vi "AdaptiveThreshold.vi"(4 "Kernel Block Size (Default: 5)":T1=enum."5", 5 "Adaptive Threshold Method":T2, 6 "Invert? (Default: False)":bool, 7 "Max Value (Default: 255)":u8=255, 8 "error in (no error)":errorcluster, 9 "C":dbl, 10 "Adaptive Threshold Result in":T3, 11 "Greyscale Image-Source in":T3) -> (0 "error out":errorcluster, 3 "Adaptive Threshold Result":T3)   [LabVIEW 2020, in "image.lvlib"]
doc: "Apply an adaptive threshold to convert a greyscale image to a binary image."
uses:
  image.lvlib
  Greyscale Image.ctl
  AdaptiveThresholdMethod.ctl
  Kernel Block Size.ctl
  common/common.lvlib
  common/bin/gartoolkit_32-1.dll
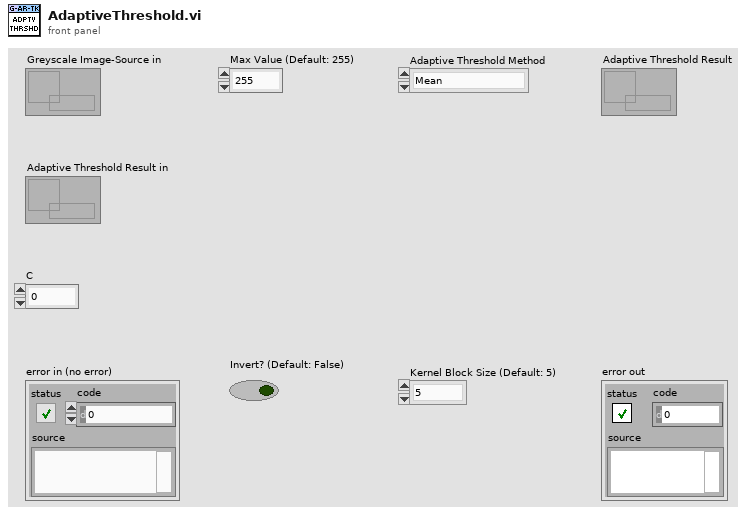
[diagram p1: front panel]
types:
  T1 = typedef "image.lvlib/Kernel Block Size.ctl" = enum16{"3", "5", "7", "9", "11", "13", "15", "17", "19", "21", "23", "25", "27", "29", "31", "33", "35", "37", "39", "41", "43", "45", "47", "49", "51", "53", "55", "57", "59", "61", "63", "65", "67", "69", "71", "73", "75", "77", "79", "81", "83", "85", "87", "89", "91", "93", "95", "97", "99", "101", "103", "105", "107", "109", "111", "113", "115", "117", "119", "121", "123", "125", "127", "129", "131", "133", "135", "137", "139", "141", "143", "145", "147", "149", "151", "153", "155", "157", "159", "161", "163", "165", "167", "169", "171", "173", "175", "177", "179", "181", "183", "185", "187", "189", "191", "193", "195", "197", "199", "201", "203", "205", "207", "209", "211", "213", "215", "217", "219", "221", "223", "225", "227", "229", "231", "233", "235", "237", "239", "241", "243", "245", "247", "249", "251", "253", "255", "257", "259", "261", "263", "265", "267", "269", "271", "273", "275", "277", "279", "281", "283", "285", "287", "289", "291", "293", "295", "297", "299", "301", "303", "305", "307", "309", "311", "313", "315", "317", "319", "321", "323", "325", "327", "329", "331", "333", "335", "337", "339", "341", "343", "345", "347", "349", "351", "353", "355", "357"}
  T2 = typedef "image.lvlib/AdaptiveThresholdMethod.ctl" = enum8{"Mean", "Gaussian"}
  T3 = typedef "image.lvlib/Greyscale Image.ctl" = refnum<data-value>
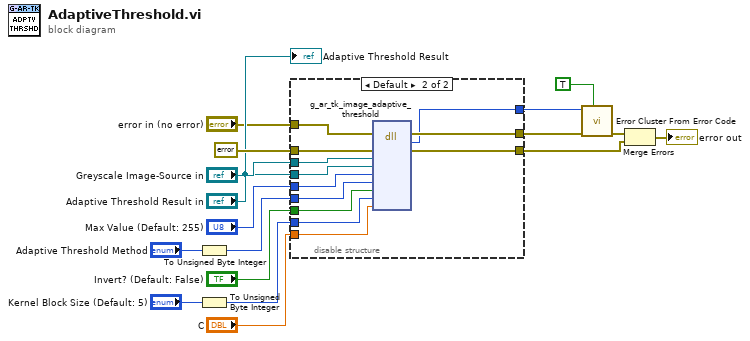
[diagram p0: block diagram]
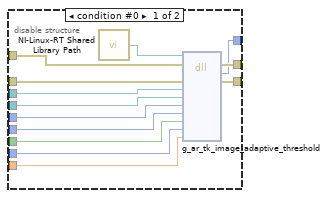
[diagram p2: hidden frame]
diagram:
  n1 = To Unsigned Byte Integer(number="Adaptive Threshold Method") -> (unsigned 8bit integer=w9:u8)
  n2 = To Unsigned Byte Integer(number="Kernel Block Size (Default: 5)") -> (unsigned 8bit integer=w7:u8)
  n3 = disable-structure shown="Default" {
    disable-tunnel: "error in (no error)" -> [w21 w42]
    disable-tunnel: errorcluster {"status"=FALSE, "code"=0, "source"=""} ("error constant") -> [w29 w41]
    disable-tunnel: "Greyscale Image-Source in" -> [w28 w40]
    disable-tunnel: "Adaptive Threshold Result in" -> [w27 w39]
    disable-tunnel: "Max Value (Default: 255)" -> [w26 w38]
    disable-tunnel: w9 -> [w25 w37]
    disable-tunnel: "Invert? (Default: False)" -> [w24 w36]
    disable-tunnel: w7 -> [w23 w35]
    disable-tunnel: "C" -> [w22 w34]
    disable-tunnel: [w20 w33] -> w5
    disable-tunnel: [w18 w32] -> w4
    disable-tunnel: [w19 w31] -> w3
    frame condition #0 {
      n4 = call "NI-Linux-RT Shared Library Path.vi"() -> ("Path"=w30:path)
      n5 = dll-call lib="?" fn="g_ar_tk_image_adaptive_threshold" ("g_ar_toolkit.*.*:g_ar_tk_image_in_range")(path in=w30, error in=w21, "error_cluster"=w29, "EDVR src"=w28, "EDVR dst"=w27, "max_value"=w26, "adaptive_method"=w25, "invert"=w24, "block_size"=w23, "c"=w22) -> (error out=w20:errorcluster, w18:i32, "error_cluster"=w19:errorcluster)  [unwired: 8 in, 1 out]
    }
    frame condition #1 (active) {
      n6 = dll-call lib="C:/serenial/lib/g-augmented-reality-toolkit/LabVIEW/common/bin/gartoolkit_*-1.*" fn="g_ar_tk_image_adaptive_threshold" ("g_ar_toolkit.*.*:g_ar_tk_image_in_range")(error in=w42, "error_cluster"=w41, "EDVR src"=w40, "EDVR dst"=w39, "max_value"=w38, "adaptive_method"=w37, "invert"=w36, "block_size"=w35, "c"=w34) -> (error out=w33:errorcluster, w32:i32, "error_cluster"=w31:errorcluster)  [unwired: 9 in, 1 out]
    }
  }
  n7 = call <vilib>:"Error Cluster From Error Code.vi"("show call chain? (False)"=TRUE, "error in (no error)"=w5, "error code (0)"=w4) -> ("error out"=w16:errorcluster)  [unwired: 6 in]
  n8 = Merge Errors(w16, w3) -> (→"error out":errorcluster)
  "Adaptive Threshold Result" <- "Adaptive Threshold Result in"
